vi "Pre Launch Init.vi"(11 "Guardar TextoPlano in":refnum<class "Guardar TextoPlano.lvclass">) -> (0 "error out":errorcluster, 3 "Guardar TextoPlano out":refnum<class "Guardar TextoPlano.lvclass">)   [LabVIEW 2020, in "Guardar TextoPlano.lvlib" / "Guardar TextoPlano.lvclass"]
doc: "(<B>Filename</B>: Actor Framework.lvlib:Actor.lvclass:Pre Launch Init.vi)\n\nDefines behavior that occurs after the Launch Nested Actor method is invoked but before the actor's Actor Core method begins running.\n\nBy default, this method does nothing. A descendant class may override it to define behavior."
uses:
  Guardar TextoPlano.lvclass
  Guardar TextoPlano.lvclass/Guardar TextoPlano.ctl
  <vilib>/ActorFramework/Actor/Actor.lvclass
panel:
  in  "Dato":string
  in  "Save?":bool
  in  "Proviene de?":enum16{"Contador", "Generador funciones"}(ring)
  in  "Exit":bool
  in  "Path":path
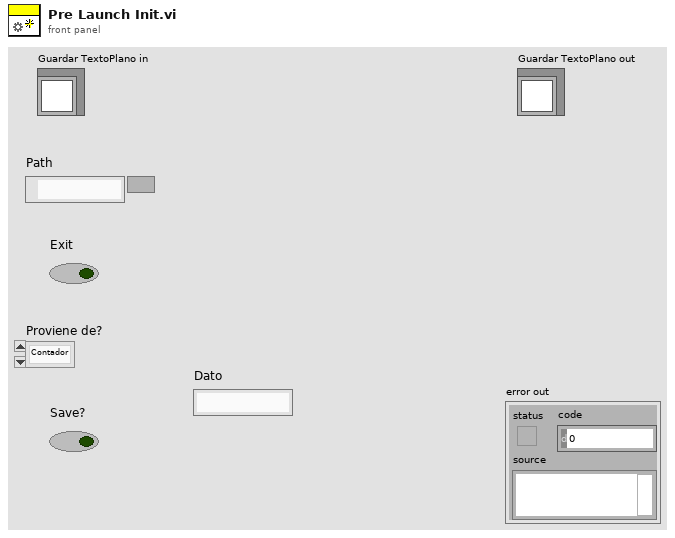
[diagram p1: front panel]
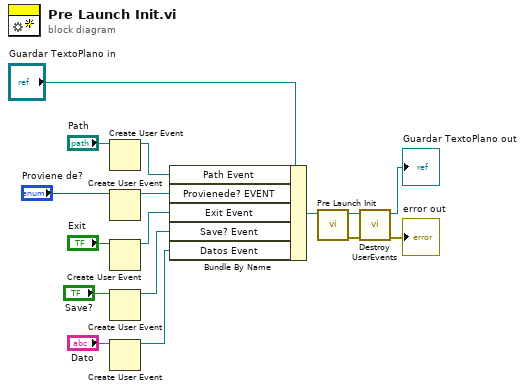
[diagram p0: block diagram]
diagram:
  n1 = Create User Event(user event datatype="Path") -> (user event=w10:refnum<user-event>)  [unwired: 1 in, 1 out]
  n2 = Create User Event(user event datatype="Proviene de?") -> (user event=w9:refnum<user-event>)  [unwired: 1 in, 1 out]
  n3 = Create User Event(user event datatype="Exit") -> (user event=w8:refnum<user-event>)  [unwired: 1 in, 1 out]
  n4 = Create User Event(user event datatype="Save?") -> (user event=w7:refnum<user-event>)  [unwired: 1 in, 1 out]
  n5 = Create User Event(user event datatype="Dato") -> (user event=w6:refnum<user-event>)  [unwired: 1 in, 1 out]
  n6 = Bundle By Name(cluster="Guardar TextoPlano in", "Path Event"=w10, "Provienede? EVENT"=w9, "Exit Event"=w8, "Save? Event"=w7, "Datos Event"=w6) -> (w5:refnum<class "Guardar TextoPlano.lvclass">)
  n7 = call-parent "Pre Launch Init.vi"("Actor in"=w5) -> ("error out"=w3:errorcluster, "Actor out"=w4:refnum<class "Guardar TextoPlano.lvclass">)  [unwired: 9 in]
  n8 = call "Destroy UserEvents.vi"("error in (no error)"=w3, "Guardar TextoPlano in"=w4) -> ("error out"=→"error out":errorcluster, "Guardar TextoPlano out"=→"Guardar TextoPlano out":refnum<class "Guardar TextoPlano.lvclass">)  [unwired: 8 in]
